vi "Test Save 2D array.vi"() -> ()   [LabVIEW 2018]
panel:
  in  "file path (use dialog)":path=path "D:/191119/test.dat"
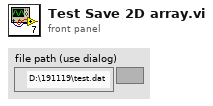
[diagram p1: front panel]
types:
  T1 = enum16{"big-endian, network order", "native, host order", "little-endian"}
  T2 = enum16{"open", "replace", "create", "open or create", "replace or create", "replace or create with confirmation"}
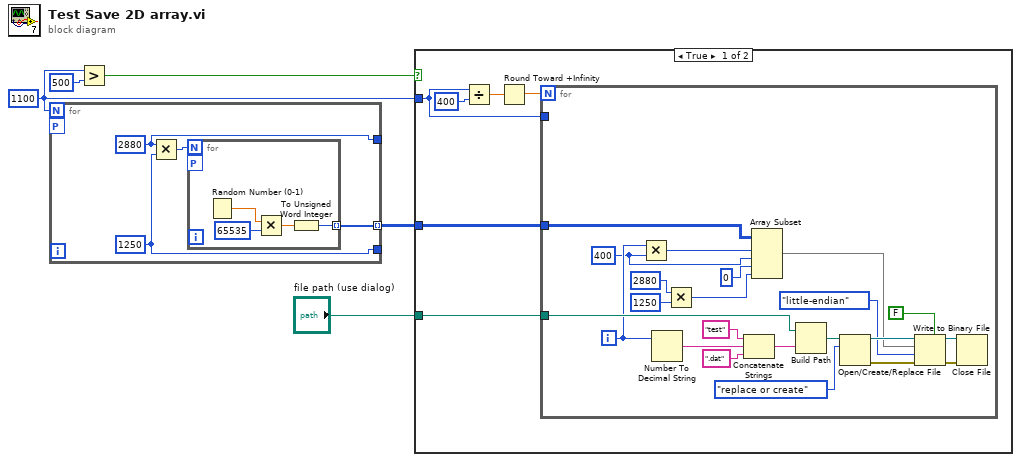
[diagram p0: block diagram]
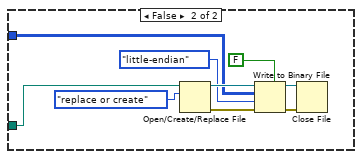
[diagram p2: hidden frame]
diagram:
  w2 = 1100
  n1 = for {
    N: w2 -> [_]
    tunnel: [w8] -> w5 mode=indexing
    tunnel: [w7] -> _
    tunnel: [w6] -> _
    workers-P: _ -> [_]
    w6 = 1250
    w7 = 2880
    n2 = Multiply(x=w7, y=w6) -> (x*y=w9:i32)
    n3 = for {
      N: w9 -> [_]
      tunnel: [w10] -> w8 mode=indexing
      workers-P: _ -> [_]
      n4 = Random Number (0-1)() -> (number: 0 to 1=w13:dbl)
      n5 = Multiply(x=w13, y=u16 65535) -> (x*y=w11:dbl)
      n6 = To Unsigned Word Integer(number=w11) -> (unsigned 16bit integer=w10:u16)
    }
  }
  n7 = Greater?(x=w2, y=500) -> (0:w3:bool)
  n8 = case shown="True" w3 {
    tunnel: w5 -> [w15 w44]
    tunnel: w2 -> [w14 _]
    tunnel: "file path (use dialog)" -> [w16 w43]
    frame True {
      n9 = Divide(x=w14, y=400) -> (x/y=w18:dbl)
      n10 = Round Toward +Infinity(x=w18) -> (ceil(x): smallest int >= x=w17:dbl)
      n11 = for {
        N: w17 -> [_]
        tunnel: w16 -> [w35]
        tunnel: w15 -> [w34]
        tunnel: w14 -> [_]
        i -> [w22]
        w20 = 400 ("y")
        n12 = Multiply(x=w22, y=w20) -> (x*y=w21:i32)
        n13 = Number To Decimal String(number=w22) -> (decimal integer string=w25:string)  [unwired: 1 in]
        n14 = Multiply(x=2880, y=1250) -> (x*y=w27:i32)
        n15 = Concatenate Strings("test" ("string"), w25, ".dat" ("string")) -> (w23:string)
        n16 = Array Subset(array=w34, index (row)=w21, length (row)=w20, index (col)=0 ("index"), length (col)=w27) -> (w32:u16[][])
        n17 = Build Path(base path=w35, name or relative path=w23) -> (appended path=w30:path)
        n18 = Open/Create/Replace File(file path (use dialog)=w30, operation (0:open)=T2."replace or create") -> (refnum out=w37:refnum<file>, error out=w39:errorcluster)  [unwired: 4 in, 1 out]
        n19 = Write to Binary File(file (use dialog)=w37, data=w32, error in=w39, 5:FALSE ("prepend array or string size? (T)"), 9:T1."little-endian" ("byte order (0:big-endian, network order)")) -> (refnum out=w36:refnum<file>, error out=w38:errorcluster)  [unwired: 1 in, 1 out]
        n20 = Close File(refnum=w36, error in=w38) -> ()  [unwired: 2 out]
      }
    }
    frame False {
      n21 = Open/Create/Replace File(file path (use dialog)=w43, operation (0:open)=T2."replace or create") -> (refnum out=w46:refnum<file>, error out=w48:errorcluster)  [unwired: 4 in, 1 out]
      n22 = Write to Binary File(file (use dialog)=w46, data=w44, error in=w48, 5:FALSE ("prepend array or string size? (T)"), 9:T1."little-endian" ("byte order (0:big-endian, network order)")) -> (refnum out=w45:refnum<file>, error out=w47:errorcluster)  [unwired: 1 in, 1 out]
      n23 = Close File(refnum=w45, error in=w47) -> ()  [unwired: 2 out]
    }
  }
